vi "BNO055 Reading Scaler.vi"(8 "Calibration":u32, 9 "LSB Divider":dbl=1.0, 10 "index":i32, 11 "AMG Reading":u8[](array[numeric])) -> (3 "Sensor Cluster":cluster{"X":dbl, "Y":dbl, "Z":dbl, "Cal":u32})   [LabVIEW 2017]
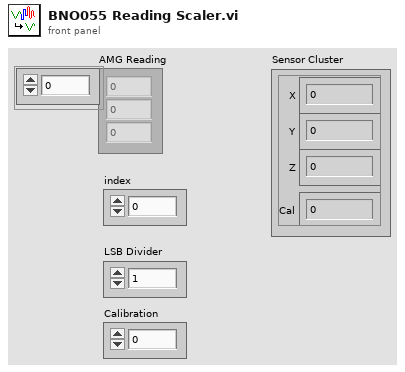
[diagram p1: front panel]
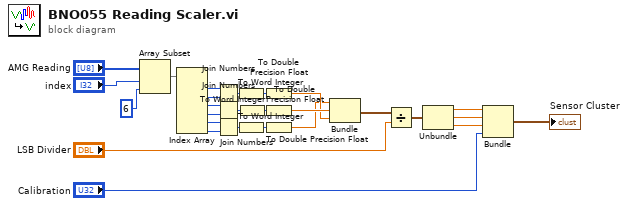
[diagram p0: block diagram]
diagram:
  n1 = Array Subset(array="AMG Reading", index="index", length=6) -> (w13:u8[])
  n2 = Index Array(array=w13) -> (element #1=w18:u8, element #2=w17:u8, element #3=w19:u8, element #4=w20:u8, element #5=w21:u8, element #6=w22:u8)  [unwired: 6 in]
  n3 = Join Numbers(hi=w18, lo=w17) -> ((hi.lo)=w12:u16)
  n4 = Join Numbers(hi=w19, lo=w20) -> ((hi.lo)=w23:u16)
  n5 = Join Numbers(hi=w21, lo=w22) -> ((hi.lo)=w24:u16)
  n6 = To Word Integer(number=w12) -> (16bit integer=w3:i16)
  n7 = To Word Integer(number=w24) -> (16bit integer=w1:i16)
  n8 = To Word Integer(number=w23) -> (16bit integer=w2:i16)
  n9 = To Double Precision Float(number=w3) -> (double precision float=w26:dbl)
  n10 = To Double Precision Float(number=w2) -> (double precision float=w27:dbl)
  n11 = To Double Precision Float(number=w1) -> (double precision float=w25:dbl)
  n12 = Bundle(w25, w27, w26) -> (w11:cluster{dbl, dbl, dbl})  [unwired: 1 in]
  n13 = Divide(x=w11, y="LSB Divider") -> (x/y=w9:cluster{dbl, dbl, dbl})
  n14 = Unbundle(w9) -> (w8:dbl, w7:dbl, w6:dbl)
  n15 = Bundle(w8, w7, w6, "Calibration"="Calibration") -> (→"Sensor Cluster":cluster{dbl, dbl, dbl, "Calibration":u32})  [unwired: 1 in]
